vi "CH_LM Error Query.vi"(0 "Meter Index":i32, 5 "error in (no error)":errorcluster, 7 "Timeout / ms (3000)":i32=3000, 9 "Lock Timeout / ms (1000)":i32=1000) -> (11 "Lock timed out":bool, 14 "Meter Index":i32, 15 "Error Code":i32[](array[numeric]), 18 "Error Message":string, 19 "error out":errorcluster)   [LabVIEW 2017, in "CH_LM.lvlib"]
doc: "Queries the instrument for any errors in the instrument's error queue. It will continue to read errors until all errors have been read from the instrument. Any errors will be returned in the <B>error out</B> control.\n\n<B>Note:</B>\nThis VI is called automatically by most driver VIs so it is not usually necessary to call this in an application."
uses:
  CH_LM.lvlib
panel:
  out "Response":string
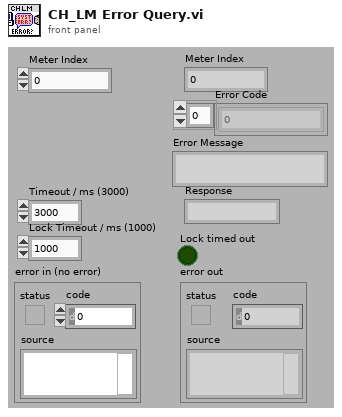
[diagram p1: front panel]
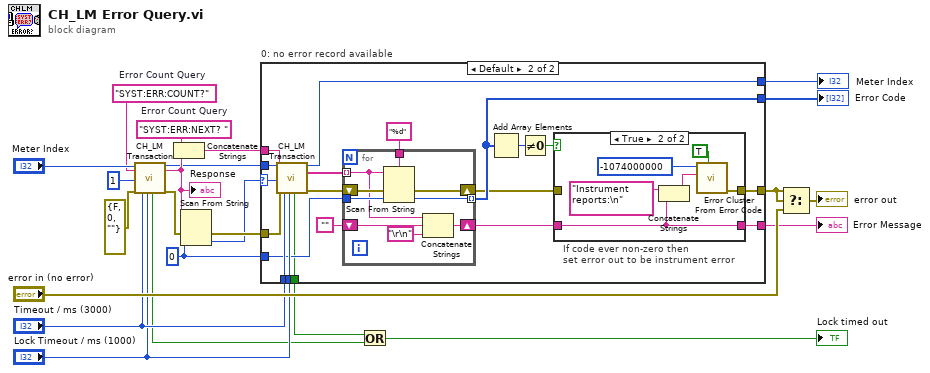
[diagram p0: block diagram]
diagram:
  w6 = 0
  w12 = "SYST:ERR:NEXT? "  # Error Count Query
  w14 = "SYST:ERR:COUNT?"  # Error Count Query
  n1 = call "CH_LM Transaction.vi"("Meter Index"="Meter Index", "Command String"=w14, "NofStrings (-1:all)"=1, "error in (no error)"=errorcluster {"status"=FALSE, "code"=0, "source"=""}, "Timeout / ms (3000)"="Timeout / ms (3000)", "Lock Timeout / ms (1000)"="Lock Timeout / ms (1000)") -> ("Lock timed out"=w3:bool, "Meter Index"=w8:i32, "Response"=w9:string, "error out"=w10:errorcluster)  [unwired: 10 out]
  "Response" <- w9
  n2 = Concatenate Strings(w12, w9) -> (w11:string)
  n3 = Scan From String(input string=w9, error in=w10, default 1=w6) -> (error out=w7:errorcluster, output 1=w1:i32)  [unwired: 2 in, 2 out]
  n4 = case "0: no error record available" shown="Default" w1 {
    selector: w1 -> [_ w26]
    tunnel: [w25 w45] -> w23
    tunnel: [_ w44] -> w19
    tunnel: [_ w43] -> w18
    tunnel: "Timeout / ms (3000)" -> [_ w42]
    tunnel: "Lock Timeout / ms (1000)" -> [_ w41]
    tunnel: w11 -> [_ w39]
    tunnel: w8 -> [w25 w38]
    tunnel: w7 -> [w24 w37]
    tunnel: w6 -> [_ w34]
    tunnel: [w24 w28] -> w5
    tunnel: [_ w27] -> w4
    frame 0 {
    }
    frame Default {
      n5 = call "CH_LM Transaction.vi"("Meter Index"=w38, "Command String"=w39, "NofStrings (-1:all)"=w26, "error in (no error)"=w37, "Timeout / ms (3000)"=w42, "Lock Timeout / ms (1000)"=w41) -> ("Lock timed out"=w27:bool, "Meter Index"=w45:i32, "Response Array"=w35:string[], "error out"=w36:errorcluster)  [unwired: 10 out]
      n6 = for {
        tunnel: w35 -> [w46] mode=indexing
        tunnel: w34 -> [w53]
        shift-right: [w52] -> w33
        shift-left: w36 -> [w54]
        tunnel: [w51] -> w43 mode=indexing
        tunnel: "%d" ("format string") -> [w50]
        shift-right: [w48] -> w29
        shift-left: "" -> [w49]
        n7 = Scan From String(format string=w50, input string=w46, error in=w54, default 1=w53) -> (error out=w52:errorcluster, output 1=w51:i32)  [unwired: 1 in, 2 out]
        n8 = Concatenate Strings(w46, w49, "\r\n") -> (w48:string)
      }
      n9 = Add Array Elements(numeric array=w43) -> (sum=w31:i32)
      n10 = Not Equal To 0?(x=w31) -> (x != 0?=w40:bool)
      n11 = case "If code ever non-zero then\nset error out to be instrument error" shown="True" w40 {
        tunnel: w29 -> [w55 w57]
        tunnel: [w56 w58] -> w28
        tunnel: w33 -> [w56 _]
        tunnel: [w55 w57] -> w44
        frame False {
        }
        frame True {
          n12 = Concatenate Strings("Instrument reports:\n" ("Source"), w57) -> (w59:string)
          n13 = call <vilib>:"Error Cluster From Error Code.vi"("show call chain? (False)"=TRUE, "error message (\"\")"=w59, "error code (0)"=-1074000000 ("Code")) -> ("error out"=w58:errorcluster)  [unwired: 1 in, 5 out]
        }
      }
    }
  }
  "Meter Index" <- w23
  "Error Message" <- w19
  "Error Code" <- w18
  n14 = Or(x=w4, y=w3) -> (x .or. y?=→"Lock timed out":bool)
  n15 = Select(t=w5, s=w5, f="error in (no error)") -> (s? t:f=→"error out":errorcluster)
